vi "MainPanel_20170525.vi"() -> (0 "ErrorOut":errorcluster)   [LabVIEW 2018] (continued)
                n229 = call "LaunchSystemMessageDialogBox.vi"("ErrorToProcess"=w547, "SMS"=w542, "ErrorIn"=w549, "CorrAct"="Undocumented System Error, please record this information and contact the vendor.", "Timeout(ms)"=-1 ("Timeout (-1)")) -> ("ErrorOut"=w548:errorcluster)  [unwired: 6 in]
              }
              frame -8998 {
                # "-1 dictates that the message box does NOT time out"
                # "Default Error Case handles all error codes undefined by this structure."
                n230 = Bundle By Name(cluster=w553, "Stat.SysState"=SystemStateEnum."System Fault") -> (w552:T29)
                n231 = Unbundle By Name(w552) -> ("SMS"=w551:T33)
                n232 = call "LaunchSystemMessageDialogBox.vi"("ErrorToProcess"=w556, "SMS"=w551, "ErrorIn"=w558, "CorrAct"="The FPGAs are configured for an external 10 MHz reference clock. It doesn't look like that clock is working right.", "Timeout(ms)"=-1 ("Timeout (-1)")) -> ("ErrorOut"=w557:errorcluster)  [unwired: 6 in]
              }
              frame 5000 {
                # "Example User Defined Error Code.  Disable the Hardware and no Dialog Box"
                n233 = Bundle By Name(cluster=w560, "Stat.SysState"=SystemStateEnum."System Fault") -> (w561:T29)
              }
              frame 5998 {
                n234 = Unbundle By Name(w565) -> ("SMS"=w568:T33)
                n235 = call "LaunchSystemMessageDialogBox.vi"("ErrorToProcess"=w567, "SMS"=w568, "ErrorIn"=w564, "CorrAct"="Error Log Failure\n\n- There was an error writing to the Error Log File, please verify that the current user has read/write permissions to the <Users>\\My Documents & the <Users>\\Desktop folders" ("CorrAction"), "Timeout(ms)"=-1) -> ("ErrorOut"=w566:errorcluster)  [unwired: 6 in]
              }
              frame 5999 {
                n236 = Bundle By Name(cluster=w572, "Stat.SysState"=SystemStateEnum."System Error") -> (w573:T29)
              }
              frame 5100..5149 {
                # "Disable Hardware?"
                # "These error codes are reserved for Config File Reads"
                n237 = Bundle By Name(cluster=w582, "Stat.SysState"=SystemStateEnum."System Fault") -> (w576:T29)
                n238 = Unbundle By Name(w576) -> ("SMS"=w575:T33)
                n239 = call "LaunchSystemMessageDialogBox.vi"("ErrorToProcess"=w579, "SMS"=w575, "ErrorIn"=w578, "CorrAct"="Configuration File Read Error\n\n- One or more Configuration File Fields were not found or improperly loaded.\n- All System Hardware has been disabled\n- Launch the Configuration Panels and verify that all values have been correctly entered\n- Reinitialize the Hardware" ("CorrAction"), "Timeout(ms)"=-1 ("Timeout")) -> ("ErrorOut"=w577:errorcluster)  [unwired: 6 in]
              }
              frame 5150..5199 {
                # "No need to disable hardware here"
                # "These error codes are reserved for Config File Writes"
                n240 = Unbundle By Name(w584) -> ("SMS"=w585:T33)
                n241 = call "LaunchSystemMessageDialogBox.vi"("ErrorToProcess"=w588, "SMS"=w585, "ErrorIn"=w587, "CorrAct"="Configuration File Write Error\n\n- One or more Configuration File Fields were not found or specified incorrectly.\n- Launch the Configuration Panels and verify that all values have been correctly entered" ("CorrAction"), "Timeout(ms)"=-1 ("Timeout")) -> ("ErrorOut"=w586:errorcluster)  [unwired: 6 in]
              }
            }
          }
        }
      }
      frame "Spvsr_Config" {
        # "Opens the Configuration Panel"
        n242 = Current VI's Path() -> (path=w595:path)
        n243 = call "SetVIWindowTransparency.vi"("VIPath"=w595, "ErrorIn"=w596) -> ("ErrorOut"=w594:errorcluster)  [unwired: 9 in]
        n244 = call "ConfigPanel.vi"("ErrorIn"=w594, "ClusterIn"=w597) -> ("ErrorOut"=w590:errorcluster, "ClusterOut"=w591:T29)  [unwired: 8 out]
        n245 = Current VI's Path() -> (path=w592:path)
        n246 = call "RestoreVIWindowTransparency.vi"("VIPath"=w592, "ErrorIn"=w590) -> ("ErrorOut"=w593:errorcluster)  [unwired: 9 in]
      }
      frame "Spvsr_FPConfig" {
        w641 = ScaleMeasure."50" ("ScaleMeasure")
        w638 = ext 1.0 ("Scale_In_RT")
        w639 = fxp<+/-,30,30> 536870911.0 ("Scale_NoiseFloor")
        # "Don't start other loops if paths are bad."
        n247 = disable-structure shown="Enabled" {
          disable-tunnel: w603 -> [w661 _]
          disable-tunnel: [w660 T38 {"#NoiseSums"=1, "Max_df"=1, "AvgAvg"=FALSE, "#Avg"=1, "AutoCenter"=FALSE, "Inclin"={"Vmin"=0.0, "Vmax"=0.0, "Angle_min"=0.0, "Angle_max"=0.0, "Offset"=0.0, "Pos_Neg"=FALSE}, "1"={"Cal_"={"Fine"=0.000213623046875, "Coarse_"=4194303.0}, "Beac"={"Fine"=4194303.0, "Coarse_"=1.0}, "Scale"={"Step4"=10000.0, "Step5"=4194303.0, "Step6"=1.0, "Step7"=10000.0}, "Offset"=0.0, "Scale_Noise"=4194303.0, "Scale_Step1"=65535.0, "Scale_In_RT"=1.0, "ScaleMeas"=0.999969482421875, "FreqsToRemove"=[0, 1633], "Width"=[0, 1633], "ScaleMeasEnum"=enum."50", "FilterEnab"=enum."Step 1"}, "2"={"Cal_"={"Fine"=0.000213623046875, "Coarse_"=4194303.0}, "Beac"={"Fine"=0.000213623046875, "Coarse_"=4194303.0}, "Scale"={"Step4"=0.0, "Step5"=4194303.0, "Step6"=1.0, "Step7"=10000.0}, "Offset"=0.0, "Scale_Noise"=4194303.0, "Scale_Step1"=65535.0, "Scale_In_RT"=1.0, "ScaleMeas"=0.999969482421875, "FreqsToRemove"=[0, 1633], "Width"=[0, 1633], "ScaleMeasEnum"=enum."50", "FilterEnab"=enum."Step 1"}, "3"={"Cal_"={"Fine"=0.000213623046875, "Coarse_"=4194303.0}, "Beac"={"Fine"=0.000213623046875, "Coarse_"=4194303.0}, "Scale"={"Step4"=0.0, "Step5"=4194303.0, "Step6"=1.0, "Step7"=10000.0}, "Offset"=0.0, "Scale_Noise"=4194303.0, "Scale_Step1"=65535.0, "Scale_In_RT"=1.0, "ScaleMeas"=0.999969482421875, "FreqsToRemove"=[0, 1633], "Width"=[0, 1633], "ScaleMeasEnum"=enum."50", "FilterEnab"=enum."Step 1"}, "4"={"Cal_"={"Fine"=0.000213623046875, "Coarse_"=4194303.0}, "Beac"={"Fine"=0.000213623046875, "Coarse_"=4194303.0}, "Scale"={"Step4"=0.0, "Step5"=4194303.0, "Step6"=1.0, "Step7"=10000.0}, "Offset"=0.0, "Scale_Noise"=4194303.0, "Scale_Step1"=1.0, "Scale_In_RT"=10000.0, "ScaleMeas"=0.999969482421875, "FreqsToRemove"=[0, 1633], "Width"=[0, 1633], "ScaleMeasEnum"=enum."50", "FilterEnab"=enum."Step 1"}, "Target to Probe"=enum."4", "SNR_Thresh"=1.0, "Paths"={"CfgFile"=path "", "LogFolder"=path "", "LogFile"=path "", "NAS path"=path "", "ThreshFile"=path "", "RedunFolder"=path ""}, "Connex_Location"="", "SimulateFPGA"=FALSE, "Deadband"=0.0} ("FP_User")] -> w602
          frame Enabled {
            # "12/14/2020"
            n248 = Unbundle By Name(w661) -> ("Config.FP_User"=w660:T38)
          }
          frame Disabled {
          }
        }
        n249 = Unbundle By Name("Scale") -> ("Measure"=w625:fxp<+/-,16,1>, "Step1"=w626:fxp<+/-,17,17>, "Scale"=w627:T4)
        n250 = call "RootExists.vi"("path"="NAS path") -> ("file or folder exists?"=w605:bool)  [unwired: 10 in]
        n251 = Negate(x="Shift Cal") -> (-x=w620:T11)
        n252 = Negate(x="Shift Beac") -> (-x=w619:T11)
        n253 = Not(x=w605) -> (.not. x?=→"Logging to NAS":bool)
        n254 = Bundle By Name(cluster=w602, "1.ScaleMeas"=w625, "1.Scale_Step1"=w626, "1.Scale"=w627, "1.ScaleMeasEnum"=w641, "AvgAvg"="AvgAvg", "1.FreqsToRemove"="FreqsToRemove", "1.Width"="Width [bins]", "1.Cal_"=w620, "1.Beac"=w619, "1.FilterEnab"="FilterEnable", "1.Scale_Noise"=w639, "1.Scale_In_RT"=w638, "AutoCenter"="AutoCenter", "Target to Probe"="Target to Probe", "#Avg"=u16 150 ("#Avg in FPGA"), "SNR_Thresh"="SNR_Thresh", "Inclin"="Inclin", "Paths.RedunFolder"="base path", "Paths.LogFolder"="base path", "Paths.NAS path"="NAS path", "Paths.ThreshFile"="ThreshFile", "Connex_Location"="Location", "Max_df"="MaxTrackRate", "SimulateFPGA"="SimulateFPGA", "Deadband"="Deadband") -> (w650:T38)
        n255 = Build Array("base path", "ThreshFile") -> (w623:path[])
        n256 = Select(t=enum32{"Auto", "Manual"}."Auto" ("FreqShiftTab"), s="AutoCenter", f=enum32{"Auto", "Manual"}."Manual" ("FreqShiftTab")) -> (s? t:f=→"FreqShiftTab_72Co" →"FreqShiftTab_84Co":enum32{"Auto", "Manual"})
        n257 = for {
          tunnel: w623 -> [w672] mode=indexing
          tunnel: [w670] -> w622 mode=indexing
          n258 = call "RootDoesntExist.vi"("base path in"=w672) -> ("String"=w671:string)  [unwired: 10 in]
          n259 = call "RootExists.vi"("path"=w672) -> ("file or folder exists?"=w670:bool)  [unwired: 10 in]
          n260 = case shown="False" w670 {
            tunnel: w671 -> [w673 _]
            frame False {
              n261 = One Button Dialog(message=w673) -> ()  [unwired: 1 in, 1 out]
            }
            frame True {
            }
          }
        }
        n262 = Unbundle By Name(w650) -> ("2"=w649:T39)
        n263 = Bundle By Name(cluster=w649, "ScaleMeas"=w625, "Scale_Step1"=w626, "Scale"=w627, "ScaleMeasEnum"=w641, "FreqsToRemove"="FreqsToRemove", "Width"="Width [bins]", "FilterEnab"="FilterEnable", "Scale_Noise"=w639, "Scale_In_RT"=w638, "Cal_"=w620, "Beac"=w619) -> (w651:T39)
        n264 = Bundle By Name(cluster=w650, "2"=w651) -> (w644:T38)
        n265 = Negate(x="Shift Cal 3") -> (-x=w618:T11)
        n266 = Negate(x="Shift Beac 3") -> (-x=w617:T11)
        n267 = Unbundle By Name(w644) -> ("3"=w648:T39)
        n268 = Bundle By Name(cluster=w648, "ScaleMeas"=w625, "Scale_Step1"=w626, "Scale"=w627, "ScaleMeasEnum"=w641, "FreqsToRemove"="FreqsToRemove 2", "Width"="Width 2 [bins]", "FilterEnab"="FilterEnable", "Scale_Noise"=w639, "Scale_In_RT"=w638, "Cal_"=w618, "Beac"=w617) -> (w647:T39)
        n269 = And Array Elements(Boolean array=w622) -> (logical AND=w621:bool)
        n270 = Bundle By Name(cluster=w644, "3"=w647) -> (w643:T38)
        n271 = Unbundle By Name(w643) -> ("4"=w645:T39)
        n272 = Bundle By Name(cluster=w645, "ScaleMeas"=w625, "Scale_Step1"=w626, "Scale"=w627, "ScaleMeasEnum"=w641, "FreqsToRemove"="FreqsToRemove 2", "Width"="Width 2 [bins]", "FilterEnab"="FilterEnable", "Scale_Noise"=w639, "Scale_In_RT"=w638, "Cal_"=w618, "Beac"=w617) -> (w646:T39)
        n273 = Bundle By Name(cluster=w643, "4"=w646) -> (w642:T38)
        n274 = Bundle By Name(cluster=w603, "Config.FP_User"=w642) -> (w613:T29)
        n275 = Bundle By Name(cluster=w613, "Config.FP_User.Max_df"=u32 1) -> (w612:T29)
        n276 = case shown="True" w621 {
          tunnel: w659 -> [w663 w669]
          tunnel: w613 -> [_ w664]
          tunnel: w657 -> [_ w668]
          tunnel: [w663 w667] -> w653
          tunnel: w652 -> [_ w666]
          tunnel: w629 -> [_ w665]
          frame False {
          }
          frame True {
            n277 = call "Send_Front_Panel_Config_to_Loops.vi"("ClusterIn"=w664, "Log_Q"=w665, "error in (no error)"=w669, "Noise_Q"=w666, "Tones_Q"=w668) -> ("error out"=w667:errorcluster)  [unwired: 6 in]
          }
        }
        n278 = call "WriteConfigFile.vi"("ErrorIn"=w653, "ClusterIn"=w612) -> ("ErrorOut"=w658:errorcluster)  [unwired: 1 in, 8 out]
        "Auto Center" <- "AutoCenter"
      }
      frame "Spvsr_AlarmCfg" {
        # "We send alarm configurations to AI and TC. The voltage and\ntemp indicators are color-coded red & yellow if there are \nalarms or wanings. These are calculated in the AI loops."
        # "We need to send the alarm configuration to the log loop because that is\nwhere we will check the alarm statuses. It's the only place where we can find\nthe data from AI, TC, TE, ADAM, and spectra."
        n279 = Unbundle By Name(w686) -> ("Config.FP_User.Paths.ThreshFile"=w685:path)
        n280 = Bundle By Name(cluster=w686, "Alarm"="AlarmSettings") -> (w689:T29)
        n281 = Flatten To XML(anything="AlarmSettings") -> (xml string=w688:string)
        n282 = call-poly <vilib>:"Write to XML File.vi"("error in (no error)"=w687, "XML Input"=w688, "XML File Path"=w685) -> ("error out"=w684:errorcluster)  [unwired: 6 in, 2 out]
        n283 = To Variant(anything="AlarmSettings") -> (Variant=w675:variant)
        n284 = To Variant(anything="AlarmSettings") -> (Variant=w679:variant)
        n285 = Bundle By Name(cluster=cluster{"Enum":T17, "Data":variant} {"Enum"=enum."Log_CfgAlarm", "Data"=variant} ("element"), "Data"=w679) -> (w680:cluster{"Enum":T17, "Data":variant})
        n286 = Bundle By Name(cluster=cluster{"Enum":T49, "Var":variant} {"Enum"=enum."AI_Alarm", "Var"=variant}, "Var"=w675) -> (w676:cluster{"Enum":T49, "Var":variant})
        n287 = Enqueue Element(queue=w682, element=w680, error in (no error)=w684) -> (error out=w683:errorcluster)  [unwired: 1 in, 2 out]
        n288 = for {
          tunnel: string[] ["AI", "TC"] ("name (unnamed)") -> [w697] mode=indexing
          tunnel: w676 -> [w690]
          n289 = Obtain Queue(max queue size (-1, unlimited)=100, name (unnamed)=w697, element data type=w690) -> (queue out=w695:refnum<queue>, error out=w696:errorcluster)  [unwired: 2 in, 1 out]
          n290 = Enqueue Element(queue=w695, element=w690, error in (no error)=w696) -> (queue out=w693:refnum<queue>, error out=w694:errorcluster)  [unwired: 1 in, 1 out]
          n291 = Release Queue(queue=w693, error in (no error)=w694) -> (error out=w692:errorcluster)  [unwired: 1 in, 2 out]
          n292 = call "PushToErrorHandler.vi"("ErrorIn"=w692, "ErrorLocation"="SendAlarmToAI_orTC") -> ()  [unwired: 5 in, 1 out]
        }
      }
      frame "Spvsr_DigitzOffs" {
        w707 = fxp<+/-,16,16> 0.0 ("fixed-point type")
        n293 = local read "84 GHz"() -> (w715:T2)
        n294 = local read "72 GHz"() -> (w716:T2)
        n295 = Unbundle By Name(w716) -> ("MeasMean0"=w712:dbl, "MeasMean1"=w710:dbl)
        n296 = Unbundle By Name(w715) -> ("MeasMean0"=w709:dbl, "MeasMean1"=w708:dbl)
        n297 = Negate(x=w712) -> (-x=w702:dbl)
        n298 = Negate(x=w710) -> (-x=w701:dbl)
        n299 = Negate(x=w709) -> (-x=w700:dbl)
        n300 = Negate(x=w708) -> (-x=w699:dbl)
        n301 = To Fixed-Point(fixed-point type=w707, number=w702) -> (fixed-point=w711:fxp<+/-,16,16>)
        "Digitizer Offset 72 Co" <- w711
        n302 = To Fixed-Point(fixed-point type=w707, number=w701) -> (fixed-point=w705:fxp<+/-,16,16>)
        "Digitizer Offset 72 X" <- w705
        n303 = To Fixed-Point(fixed-point type=w707, number=w700) -> (fixed-point=w704:fxp<+/-,16,16>)
        "Digitizer Offset 84 Co" <- w704
        n304 = To Fixed-Point(fixed-point type=w707, number=w699) -> (fixed-point=w703:fxp<+/-,16,16>)
        "Digitizer Offset 84 x" <- w703
        n305 = Bundle By Name(cluster=w713, "Config.FP_User.1.Offset"=w711, "Config.FP_User.2.Offset"=w705, "Config.FP_User.3.Offset"=w704, "Config.FP_User.4.Offset"=w703) -> (w714:T29)
      }
      frame "FP_AO_ctrl" {
        w739 = 5.0
        w740 = 0.0
        w734 = cluster{"Enum":T51, "Data":variant} {"Enum"=enum."AO_Write", "Data"=variant}
        # "As defined in Wiring_Pinout Diagrams_DRAFT_20171207.xlsx\nfrom Nick Tarasenko.\nLuke 12-12-2017"
        # "Cal tones: 5 is on, 0 is off"
        # "Noise: 0 is on, 5 is off"
        n306 = Select(t=w740, s="noise_ctrl", f=w739) -> (s? t:f=w738:dbl)
        n307 = Select(t=w739, s="72GHz_ctrl", f=w740) -> (s? t:f=w737:dbl)
        n308 = Select(t=w739, s="84GHz_ctrl", f=w740) -> (s? t:f=w736:dbl)
        n309 = Obtain Queue(max queue size (-1, unlimited)=100, name (unnamed)="AO", element data type=w734, error in (no error)=w741) -> (queue out=w744:refnum<queue>, error out=w730:errorcluster)  [unwired: 1 in, 1 out]
        n310 = Build Array("noise_ctrl", "72GHz_ctrl", "84GHz_ctrl") -> (w719:bool[])
        n311 = Build Array(w738, w737, w736) -> (w735:dbl[])
        n312 = To Variant(anything=w735) -> (Variant=w723:variant)
        n313 = Bundle By Name(cluster=w734, "Data"=w723) -> (w733:cluster{"Enum":T51, "Data":variant})
        n314 = Enqueue Element(queue=w744, element=w733, error in (no error)=w730) -> (queue out=w729:refnum<queue>, error out=w731:errorcluster)  [unwired: 1 in, 1 out]
        n315 = To Variant(anything=w719) -> (Variant=w718:variant)
        n316 = Release Queue(queue=w729, error in (no error)=w731) -> (error out=w728:errorcluster)  [unwired: 1 in, 2 out]
        n317 = Bundle By Name(cluster=cluster{"Enum":T17, "Data":variant} {"Enum"=enum."Log_DO", "Data"=variant} ("element"), "Data"=w718) -> (w724:cluster{"Enum":T17, "Data":variant})
        n318 = Enqueue Element(queue=w726, element=w724, timeout in ms (-1)=10, error in (no error)=w728) -> (error out=w727:errorcluster)  [unwired: 2 out]
      }
      frame "Spvsr_ScaleGraphs" {
        w776 = 1000000.0 ("y")
        w773 = 10.0 ("y")
        n319 = local read "BeaconShift 3"() -> (w757:dbl)
        n320 = local read "BeaconShift 2"() -> (w789:dbl)
        n321 = local read "BeaconShift 4"() -> (w755:dbl)
        n322 = local read "BeaconShift"() -> (w785:dbl)
        n323 = local read "Peak Location Beacon"() -> (w771:dbl)
        n324 = local read "Peak Location Cal"() -> (w772:dbl)
        n325 = local read "Peak Location Beacon 2"() -> (w791:dbl)
        n326 = local read "Peak Location Cal 2"() -> (w792:dbl)
        n327 = local read "Peak Location Beacon 3"() -> (w753:dbl)
        n328 = local read "Peak Location Cal 3"() -> (w752:dbl)
        n329 = local read "Peak Location Beacon 4"() -> (w751:dbl)
        n330 = local read "Peak Location Cal 4"() -> (w750:dbl)
        n331 = local read "CalShift 3"() -> (w756:dbl)
        n332 = local read "CalShift 2"() -> (w790:dbl)
        n333 = local read "CalShift"() -> (w786:dbl)
        n334 = local read "CalShift 4"() -> (w754:dbl)
        n335 = control-ref of="NoiseFloor"() -> (w749:refnum<vi>)
        n336 = control-ref of="NoiseFloor 2"() -> (w747:refnum<vi>)
        n337 = control-ref of="NoiseFloor 3"() -> (w746:refnum<vi>)
        n338 = control-ref of="NoiseFloor 4"() -> (w745:refnum<vi>)
        n339 = local read "df (Hz)"() -> (w767:dbl)
        n340 = Build Array(w785, w786, w789, w790, w757, w756, w755, w754) -> (w780:dbl[])
        n341 = Build Array(w749, w747, w746, w745) -> (w748:refnum<vi>[])
        n342 = for {
          tunnel: [w820] -> w763
          tunnel: w780 -> [w822] mode=indexing
          tunnel: [w818] -> w762 mode=indexing
          n343 = local read "df (Hz)"() -> (w823:dbl)
          n344 = Divide(x=w823, y=1000000.0) -> (x/y=w820:dbl)
          n345 = Divide(x=w822, y=1000000.0) -> (x/y=w818:dbl)
        }
        n346 = Build Array(w771, w772, w791, w792, w753, w752, w751, w750) -> (w781:dbl[])
        n347 = for {
          tunnel: w767 -> [w795]
          tunnel: u8 0 ("Noise Floor") -> [w794]
          tunnel: w748 -> [w793] mode=indexing
          n348 = property class="WFGraph (strict)"(reference=w793, "YScale.Mapping Mode"=w794, "XScale.Multiplier"=w795) -> ()  [unwired: 1 in, 2 out]
        }
        n349 = case shown="True" "AutoScale Y Noise" {
          tunnel: w748 -> [_ w796]
          frame False {
          }
          frame True {
            n350 = for {
              tunnel: w796 -> [w798] mode=indexing
              n351 = property class="WFGraph (strict)"(reference=w798, "YScale.ScaleFit"=u8 1 ("Y Scale.Scale Fit")) -> ()  [unwired: 1 in, 2 out]
            }
          }
        }
        n352 = Add(x=w781, y=w773) -> (x+y=w774:dbl[])
        n353 = Subtract(x=w781, y=w773) -> (x-y=w775:dbl[])
        n354 = Divide(x=w774, y=w776) -> (x/y=w778:dbl[])
        n355 = Divide(x=w775, y=w776) -> (x/y=w779:dbl[])
        n356 = control-ref of="Beacon 2"() -> (w787:refnum<vi>)
        n357 = control-ref of="Cal 2"() -> (w788:refnum<vi>)
        n358 = control-ref of="Beacon 3"() -> (w761:refnum<vi>)
        n359 = control-ref of="Beacon"() -> (w770:refnum<vi>)
        n360 = control-ref of="Cal"() -> (w768:refnum<vi>)
        n361 = control-ref of="Cal 3"() -> (w760:refnum<vi>)
        n362 = control-ref of="Cal 4"() -> (w758:refnum<vi>)
        n363 = control-ref of="Beacon 4"() -> (w759:refnum<vi>)
        n364 = Build Array(w770, w768, w787, w788, w761, w760, w759, w758) -> (w782:refnum<vi>[])
        n365 = for {
          tunnel: w782 -> [w827] mode=indexing
          tunnel: u8 0 ("Tones") -> [w826]
          tunnel: w763 -> [w825]
          tunnel: w762 -> [w824] mode=indexing
          n366 = property class="WFGraph"(reference=w827, "YScale.Mapping Mode"=w826, "XScale.Multiplier"=w825, "XScale.Offset"=w824) -> ()  [unwired: 1 in, 2 out]
        }
        n367 = for {
          tunnel: w782 -> [w806] mode=indexing
          tunnel: "Zoom On Peak" -> [w805]
          tunnel: w778 -> [w804] mode=indexing
          tunnel: w779 -> [w803] mode=indexing
          tunnel: [w802] -> _
          n368 = case shown="True" w805 {
            tunnel: w806 -> [w811 w813]
            tunnel: w804 -> [w809 _]
            tunnel: w803 -> [w808 _]
            tunnel: [w807 w812] -> w802
            frame True {
              n369 = property class="WFGraph"(reference=w811, "XScale.ScaleFit"=u8 0 ("X Scale.Scale Fit"), "XScale.Maximum"=w809, "XScale.Minimum"=w808) -> (error out=w807:errorcluster)  [unwired: 1 in, 1 out]
            }
            frame False {
              n370 = disable-structure shown="Disabled" {
                disable-tunnel: w813 -> [w816 _]
                disable-tunnel: [w814 errorcluster {"status"=FALSE, "code"=0, "source"=""} ("error out")] -> w812
                frame Enabled {
                  n371 = property class="WFGraph"(reference=w816, "XScale.ScaleFit"=u8 2 ("X Scale.Scale Fit")) -> (error out=w814:errorcluster)  [unwired: 1 in, 1 out]
                }
                frame Disabled {
                }
              }
            }
          }
        }
        n372 = case shown="True" "AutoScale Y Tones" {
          tunnel: w782 -> [_ w799]
          frame False {
          }
          frame True {
            n373 = for {
              tunnel: w799 -> [w800] mode=indexing
              n374 = property class="WFGraph"(reference=w800, "YScale.ScaleFit"=u8 1 ("Y Scale.Scale Fit")) -> ()  [unwired: 1 in, 2 out]
            }
          }
        }
      }
      frame "Spvsr_TrackRate" {
        n375 = Bundle By Name(cluster=w829, "Stat.TrackRate"=FALSE) -> (w830:T29)
      }
      frame "Spvsr_AutoCenter" {
        w832 = FALSE  # Stat.AutoCentr
        n376 = Bundle By Name(cluster=w833, "Stat.AutoCentr"=w832) -> (w834:T29)
      }
      frame "Spvsr_RestartWarn" {
        n377 = One Button Dialog(message="When changing file paths, the change will not be implemented until the program is restarted.\n\nWhen changing the \"Connex Location\", the change will not be written to the data log header until a new file is made (either at midnight, or upon restarting.)") -> ()  [unwired: 1 in, 1 out]
      }
      frame "Spvsr_ChkTime" {
        # "Reset peak tracker to default 10 minutes after user changes it."
        # "Variable is updated in Log_TCP"
        n378 = Unbundle By Name(w854) -> ("Stat.AutoCentr"=w846:bool, "Stat.TrackRate"=w856:bool)
        n379 = call "Elapsed Time4"("Time Target (s)"=600.0, "Reset"=w856, "error in (no error)"=w857) -> ("Elapsed Time (s)"=w852:dbl, "Time has Elapsed"=w855:bool, "error out"=w853:errorcluster)  [unwired: 9 in, 5 out]
        n380 = case shown="True" w855 {
          tunnel: w854 -> [w875 w883]
          tunnel: [w875 w882] -> w843
          tunnel: w853 -> [w876 w880]
          tunnel: [w876 w877] -> w845
          tunnel: w852 -> [_ _]
          frame False {
          }
          frame True {
            n381 = control-ref of="MaxTrackRate"() -> (w879:refnum<vi>)
            n382 = property class="DigNum (strict)"(reference=w879, error in=w880, "Val(Sgnl)"=u32 1 ("Value (Signaling)")) -> (error out=w877:errorcluster)  [unwired: 1 out]
            n383 = Bundle By Name(cluster=w883, "Stat.TrackRate"=TRUE) -> (w882:T29)
          }
        }
        n384 = call "Elapsed Time5"("Time Target (s)"=600.0, "Reset"=w846, "error in (no error)"=w845) -> ("Elapsed Time (s)"=w849:dbl, "Time has Elapsed"=w847:bool, "error out"=w848:errorcluster)  [unwired: 9 in, 5 out]
        n385 = case shown="True" w847 {
          tunnel: w843 -> [w866 w874]
          tunnel: [w866 w873] -> w842
          tunnel: w848 -> [w867 w871]
          tunnel: [w867 w869] -> w844
          tunnel: w849 -> [_ _]
          frame False {
          }
          frame True {
            n386 = control-ref of="AutoCenter"() -> (w870:refnum<vi>)
            n387 = property class="Bool (strict)"(reference=w870, error in=w871, "Val(Sgnl)"=TRUE ("Value (Signaling)")) -> (error out=w869:errorcluster)  [unwired: 1 out]
            n388 = Bundle By Name(cluster=w874, "Stat.AutoCentr"=TRUE ("Stat.TrackRate")) -> (w873:T29)
          }
        }
        n389 = shared-variable ".\\Connex_Variables.lvlib\\TCP_Status"() -> (→"TCP Connection":bool)  [unwired: 1 in, 1 out]
        n390 = call "Elapsed Time3"("Time Target (s)"=2.0, "error in (no error)"=w844) -> ("Time has Elapsed"=w863:bool, "error out"=w840:errorcluster)  [unwired: 10 in, 6 out]
        n391 = Select(t=cluster{"QElmnt":T44, "Data":variant}[] [{"QElmnt"=enum."Spvsr_ScaleGraphs", "Data"=variant}, {"QElmnt"=enum."Spvsr_ChkTime", "Data"=variant}], s=w863, f=cluster{"QElmnt":T44, "Data":variant}[] [{"QElmnt"=enum."Spvsr_ChkTime", "Data"=variant}]) -> (s? t:f=w865:cluster{"QElmnt":T44, "Data":variant}[])
        n392 = for {
          tunnel: w865 -> [w886] mode=indexing
          tunnel: w864 -> [w885]
          shift-right: [w884] -> w860
          shift-left: _ -> [_]
          n393 = Enqueue Element(queue=w885, element=w886) -> (error out=w884:errorcluster)  [unwired: 2 in, 2 out]
        }
        n394 = Wait Until Next ms Multiple(millisecond multiple=u32 100 ("milliseconds to wait")) -> ()  [unwired: 1 out]
        n395 = Merge Errors(w860, w840) -> (w841:errorcluster)
      }
      frame "Spvsr_About" {
        # "Pops up the About dialog box where you can enter version, customer, contact and any other information regarding the application."
        n396 = call "About.vi"("error in"=w890, "Timeout (ms)"=5000) -> ("error out"=w889:errorcluster)  [unwired: 9 out]
      }
      frame "Spvsr_Exit" {
        # "With the Exit Button, we exit this loop and push the HW Loops to close."
        n397 = call "Exit_All_Loops.vi"("error in (no error)"=w892, "10Hz_Q"=w891, "Noise_Q"=w894, "Tones_Q"=w895) -> ("error out"=w893:errorcluster)  [unwired: 7 in]
      }
    }
    "SPVSR_Count" <- w285
  }
  n398 = call "PXI_Health_Loop.vi"("error in (no error)"=w1) -> ("error out"=w117:errorcluster)  [unwired: 10 in]
  n399 = while {
    tunnel: w77 -> [w899]
    tunnel: w100 -> [w909]
    tunnel: [w903] -> w137
    shift-right: [w902] -> _
    shift-left: T20 {"Alarms"={"Green"=FALSE, "Rx_Yell"=FALSE, "Cx_Yell"=FALSE, "Red"=FALSE, "Source"=""}, "Spectrum 1"=[], "Spectrum 2"=[], "Spectrum 3"=[], "Spectrum 4"=[], "HistoryWeighting"=0.0, "NoiseFloorSums"={"1"=0.0, "2"=0.0, "3"=0.0, "4"=0.0}, "PwrHist"={"72Co"={"Cal"=0.0, "Cal Smooth"=0.0, "Beac"=0.0, "Beac Smooth"=0.0, "NoiseFloorSum"=0.0, "NoiseFloorSum Smooth"=0.0}, "72X"={"Cal"=0.0, "Cal Smooth"=0.0, "Beac"=0.0, "Beac Smooth"=0.0, "NoiseFloorSum"=0.0, "NoiseFloorSum Smooth"=0.0}, "84Co"={"Cal"=0.0, "Cal Smooth"=0.0, "Beac"=0.0, "Beac Smooth"=0.0, "NoiseFloorSum"=0.0, "NoiseFloorSum Smooth"=0.0}, "84X"={"Cal"=0.0, "Cal Smooth"=0.0, "Beac"=0.0, "Beac Smooth"=0.0, "NoiseFloorSum"=0.0, "NoiseFloorSum Smooth"=0.0}}} -> [w901]
    i -> [w900]
    stop <- w904 stop-if-true
    # "Front panel updates"
    n400 = call "PushToErrorHandler.vi"("ErrorIn"=w909, "ErrorLocation"="FP") -> ("ErrorOut"=w911:errorcluster)  [unwired: 5 in]
    n401 = Get Queue Status(queue=w899) -> (# elements in queue=→"# in FP queue":i32)  [unwired: 2 in, 7 out]
    n402 = Dequeue Element(queue=w899, error in (no error)=w911) -> (queue out=w905:refnum<queue>, element=w910:cluster{"Enum":T26, "Data":variant}, error out=w906:errorcluster)  [unwired: 1 in, 1 out]
    n403 = Unbundle(w910) -> ("Enum"=w908:T26, "Data"=w907:variant)
    n404 = case shown="\"FP_Tone\"" w908 {
      tunnel: w907 -> [_ _ w930 w1074 w1123 w1133 w1153 w1164 _ w1251 _]
      tunnel: w906 -> [w916 w918 w923 w1075 w1125 w1135 w1155 w1165 w1180 w1252 w1264]
      tunnel: w905 -> [_ _ w921 _ _ _ _ _ _ _ w1265]
      tunnel: [_ _ _ _ _ _ _ _ _ _ TRUE] -> w904
      tunnel: [w916 w918 w923 w1075 w1126 w1134 w1154 w1159 w1180 w1240 w1263] -> w903
      tunnel: [w917 w919 w924 w1068 w1112 w1127 w1146 w1160 w1179 w1181 w1262] -> w902
      tunnel: w901 -> [w917 w919 w925 w1069 w1112 w1127 w1146 w1160 w1179 w1181 w1262]
      frame "FP_Init", Default {
        w915 = cluster{dbl, dbl, dbl}[] [] ("History Data")
        n405 = control-ref of="Freq History 84 Co"() -> (w913:refnum<vi>)
        n406 = control-ref of="Freq History 72 Co"() -> (w914:refnum<vi>)
        n407 = property class="WFChart (strict)"(reference=w914, "History Data"=w915) -> ()  [unwired: 1 in, 2 out]
        n408 = property class="WFChart (strict)"(reference=w913, "History Data"=w915) -> ()  [unwired: 1 in, 2 out]
      }
      frame "FP_Scale" {
      }
      frame "FP_Tone" {
        # "From Data_Send"
        n409 = local read "SNR_Thresh"() -> (w920:dbl)
        n410 = local read "AutoCenter"() -> (w922:bool)
        n411 = Variant To Data(error in=w923, type=cluster{"Target":T16, "1":T52} {"Target"=enum."1", "1"={"Cal"={"Shift_"=0.0, "Peak_ToFPGA"=-24999462.633451957, "MaxValue"=0.0, "MaxIndex"=0, "Tone"={"PkLocTrak"=0.0, "PkLocDisp"=0.0, "df_"=0.0, "ZoomPwr"=[], "Phase"=0.0, "PhaseOld"=0.0, "AboveThresh?"=FALSE, "MaxI"=0.0, "MaxQ"=0.0, "median"=0.0, "ISpect"=[], "QSpect"=[], "DeltaPhase"=0.0}, "TimeDomainI"=[], "TimeDomainQ"=array[12500 elements], "PwrSpectrum"=[], "RunningAvgFreq"=0.0, "ISpectPos"=[], "ISpectNeg"=[], "QSpectPos"=[], "QSpectNeg"=[], "10Hz_PwrSpectr"=[], "SNR"=0.0, "AliasWarn"=FALSE, "10Hz_Peak"=[], "ISpect+-"=[], "QSpect+-"=[], "TimeStamp"=timestamp(0 s since 1904-01-01), "I_Index"=array[12500 elements], "Q_Index"=array[12500 elements], "10MHz"=FALSE}, "Beac"={"Shift_"=0.0, "Peak_ToFPGA"=-24999462.633451957, "MaxValue"=0.0, "MaxIndex"=0, "Tone"={"PkLocTrak"=0.0, "PkLocDisp"=0.0, "df_"=0.0, "ZoomPwr"=[], "Phase"=0.0, "PhaseOld"=0.0, "AboveThresh?"=FALSE, "MaxI"=0.0, "MaxQ"=0.0, "median"=0.0, "ISpect"=[], "QSpect"=[], "DeltaPhase"=0.0}, "TimeDomainI"=[], "TimeDomainQ"=array[12500 elements], "PwrSpectrum"=[], "RunningAvgFreq"=0.0, "ISpectPos"=[], "ISpectNeg"=[], "QSpectPos"=[], "QSpectNeg"=[], "10Hz_PwrSpectr"=[], "SNR"=0.0, "AliasWarn"=FALSE, "10Hz_Peak"=[], "ISpect+-"=[], "QSpect+-"=[], "TimeStamp"=timestamp(0 s since 1904-01-01), "I_Index"=array[12500 elements], "Q_Index"=array[12500 elements], "10MHz"=FALSE}, "Time"=[], "Saturat"={"MeasMean0"=0.0, "MeasMean1"=0.0, "MeasMax"=0.0, "1_Max"=0.0, "4_Max"=0.0, "5_Max"=0.0, "6_Max"=0.0, "7_Max"=0.0}}} ("cluster"), Variant=w930) -> (data=w928:cluster{"Target":T16, "1":T52})  [unwired: 1 out]
        n412 = Unbundle(w928) -> ("Target"=w927:T16, "1"=w926:T52)
        n413 = case shown="\"2\", Default" w927 {
          tunnel: w926 -> [w970 w997 w1035 w1064]
          tunnel: w925 -> [w960 w985 w1021 w1051]
          tunnel: [w961 w989 w1028 w1057] -> w924
          tunnel: w922 -> [w956 _ w1024 _]
          tunnel: w921 -> [_ _ _ w1038]
          tunnel: w920 -> [w946 _ w1017 _]
          frame "1" {
            # "Reset\nWatchdog"
            # "Update all history charts"
            # "All freq locations displayed as positive."
            # "df is the same for cal & beac"
            n414 = Unbundle By Name(w970) -> ("Cal"=w969:T53, "Saturat"=→"72 GHz":T2, "Beac"=w967:T53)
            n415 = Unbundle By Name(w967) -> ("Shift_"=w966:dbl, "MaxValue"=w954:dbl, "Tone"=w945:T54, "TimeDomainI"=→"TimeDomainBeac 72Co":ext[], "PwrSpectrum"=w948:dbl[], "SNR"=→"SNR":dbl)
            "Channel Power Beac" <- w954
            n416 = Unbundle By Name(w969) -> ("Shift_"=w968:dbl, "MaxValue"=w941:dbl, "Tone"=w952:T54, "TimeDomainI"=→"TimeDomainCal 72Co":ext[], "PwrSpectrum"=→"Cal":dbl[])
            "Channel Power Cal" <- w941
            "MaxValue_Cal_72Co" <- w941
            n417 = Unbundle By Name(w945) -> ("PkLocDisp"=w964:dbl)
            n418 = Negate(x=w968) -> (-x=w942:dbl)
            "CalShift" <- w942
            n419 = Negate(x=w966) -> (-x=w944:dbl)
            "BeaconShift" <- w944
            n420 = Unbundle By Name(w952) -> ("PkLocTrak"=w965:dbl, "df_"=→"df (Hz)":dbl)
            n421 = Negate(x=w964) -> (-x=w943:dbl)
            "Peak Location Beacon" <- w943
            n422 = Unbundle By Name(w945) -> ("median"=w949:dbl, "Phase"=→"72 Co Beac":dbl)
            n423 = Negate(x=w965) -> (-x=w934:dbl)
            "Peak Location Cal" <- w934
            n424 = call "CombineSpectrumAndMedian.vi"("SNR_Thresh"=w946, "median"=w949, "PwrSpectrum"=w948) -> ("Array"=→"Beacon":dbl[][])  [unwired: 8 in]
            n425 = Bundle(w934, w943, w944) -> (→"Freq History 72 Co":cluster{dbl, dbl, dbl})  [unwired: 1 in]
            n426 = local read "NoiseFloorSum"() -> (w959:dbl)
            n427 = Divide(x=w934, y=1000000.0 ("x")) -> (x/y=→"72CoCalFrq":dbl)
            n428 = Divide(x=w943, y=1000000.0 ("x")) -> (x/y=→"72CoBeacFrq":dbl)
            n429 = call "BuildHistoryCluster.vi"("NewValueWeighting"="NewValueWeighting", "NoiseFloorSum"=w959, "Channel Power Beac"=w954, "Channel Power Cal"=w941) -> ("output cluster"=w933:T68)  [unwired: 7 in]
            n430 = control-ref of="Shift Beac"() -> (w957:refnum<vi>)
            n431 = control-ref of="Shift Cal"() -> (w958:refnum<vi>)
            n432 = Bundle By Name(cluster=w960, "Spectrum 1"=w948, "HistoryWeighting"="NewValueWeighting", "PwrHist.72Co"=w933) -> (w961:T20)
            n433 = call "OverWriteManualShiftValues.vi"("AutoCenter"=w956, "Shift Beac Val"=w944, "Shift Beac Ref"=w957, "Shift Cal Val"=w942, "Shift Cal Ref"=w958) -> ()  [unwired: 7 in]
            n434 = call "Watchdog_Functional_Global.vi"("Watchdog"=WatchdogTimer_Enum."FP") -> ()  [unwired: 8 in, 3 out]
          }
          frame "2", Default {
            n435 = Unbundle By Name(w997) -> ("Cal"=w996:T53, "Beac"=w995:T53)
            n436 = Unbundle By Name(w995) -> ("Shift_"=w994:dbl, "MaxValue"=w987:dbl, "Tone"=w982:T54, "TimeDomainI"=→"TimeDomainBeacon 72 X":ext[], "PwrSpectrum"=w988:dbl[], "SNR"=→"SNR 2":dbl, "Tone.DeltaPhase"=→"Delta Phase 72 GHz":dbl)
            "Beacon 2" <- w988
            "Channel Power Beac 2" <- w987
            n437 = Unbundle By Name(w996) -> ("Shift_"=w993:dbl, "MaxValue"=w974:dbl, "Tone"=w983:T54, "TimeDomainI"=→"TimeDomainCal 72 X":ext[], "PwrSpectrum"=→"Cal 2":dbl[])
            "Channel Power Cal 2" <- w974
            "MaxValue_Cal_72X" <- w974
            n438 = Unbundle By Name(w983) -> ("PkLocTrak"=w991:dbl)  [unwired: 1 out]
            n439 = Negate(x=w993) -> (-x=→"CalShift 2":dbl)
            n440 = Unbundle By Name(w982) -> ("PkLocDisp"=w992:dbl)
            n441 = Negate(x=w994) -> (-x=→"BeaconShift 2":dbl)
            n442 = Unbundle By Name(w982) -> ("Phase"=→"72 X Beac":dbl)
            n443 = Negate(x=w991) -> (-x=→"Peak Location Cal 2":dbl)
            n444 = Negate(x=w992) -> (-x=→"Peak Location Beacon 2":dbl)
            n445 = Unbundle By Name(w985) -> ("HistoryWeighting"=w984:dbl)
            n446 = local read "NoiseFloorSum 2"() -> (w986:dbl)
            n447 = call "BuildHistoryCluster.vi"("NewValueWeighting"=w984, "NoiseFloorSum"=w986, "Channel Power Beac"=w987, "Channel Power Cal"=w974) -> ("output cluster"=w971:T68)  [unwired: 7 in]
            n448 = Bundle By Name(cluster=w985, "Spectrum 2"=w988, "PwrHist.72X"=w971) -> (w989:T20)
          }
          frame "3" {
            # "Disdrometer device resets every 90 days UNLESS signal is too low. Using a variable\nbecause there is no other mechanism for sending data to Disdrometer"
            n449 = Unbundle By Name(w1035) -> ("Cal"=w1034:T53, "Saturat"=→"84 GHz":T2, "Beac"=w1010:T53)
            n450 = Unbundle By Name(w1010) -> ("Shift_"=w1033:dbl, "MaxValue"=w1023:dbl, "Tone"=w1014:T54, "TimeDomainI"=→"TimeDomain Beac 84 Co":ext[], "PwrSpectrum"=w1018:dbl[], "SNR"=w1012:dbl)
            "Channel Power Beac 3" <- w1023
            "SNR 3" <- w1012
            n451 = Unbundle By Name(w1034) -> ("Shift_"=w1032:dbl, "MaxValue"=w1011:dbl, "Tone"=w1019:T54, "TimeDomainI"=→"TimeDomainCal 84 Co":ext[], "PwrSpectrum"=→"Cal 3":dbl[])  [unwired: 1 out]
            "Channel Power Cal 3" <- w1011
            "MaxValue_Cal_84Co" <- w1011
            n452 = Unbundle By Name(w1014) -> ("PkLocDisp"=w1031:dbl)
            n453 = Unbundle By Name(w1014) -> ("Phase"=→"84 Co Beac":dbl, "median"=w1016:dbl)
            n454 = Unbundle By Name(w1019) -> ("PkLocTrak"=w1030:dbl)  [unwired: 1 out]
            n455 = Negate(x=w1033) -> (-x=w1013:dbl)
            "BeaconShift 3" <- w1013
            n456 = Negate(x=w1032) -> (-x=w1027:dbl)
            "CalShift 3" <- w1027
            n457 = Negate(x=w1031) -> (-x=w1004:dbl)
            "Peak Location Beacon 3" <- w1004
            n458 = Negate(x=w1030) -> (-x=w1002:dbl)
            "Peak Location Cal 3" <- w1002
            n459 = shared-variable ".\\Disdrometer_Vars.lvlib\\Disdrom_SNR"(w1012) -> ()  [unwired: 1 in, 1 out]
            n460 = Divide(x=w1002, y=1000000.0 ("x")) -> (x/y=→"84CoCalFrq":dbl)
            n461 = call "CombineSpectrumAndMedian.vi"("SNR_Thresh"=w1017, "median"=w1016, "PwrSpectrum"=w1018) -> ("Array"=→"Beacon 3":dbl[][])  [unwired: 8 in]
            n462 = Divide(x=w1004, y=1000000.0 ("x")) -> (x/y=→"84CoBeacFrq":dbl)
            n463 = Bundle(w1002, w1004, w1013) -> (→"Freq History 84 Co":cluster{dbl, dbl, dbl})  [unwired: 1 in]
            n464 = local read "NoiseFloorSum 2"() -> (w1022:dbl)
            n465 = Unbundle By Name(w1021) -> ("HistoryWeighting"=w1020:dbl)
            n466 = call "BuildHistoryCluster.vi"("NewValueWeighting"=w1020, "NoiseFloorSum"=w1022, "Channel Power Beac"=w1023, "Channel Power Cal"=w1011) -> ("output cluster"=w999:T68)  [unwired: 7 in]
            n467 = control-ref of="Shift Cal 3"() -> (w1026:refnum<vi>)
            n468 = control-ref of="Shift Beac 3"() -> (w1025:refnum<vi>)
            n469 = Bundle By Name(cluster=w1021, "Spectrum 3"=w1018, "PwrHist.84Co"=w999) -> (w1028:T20)
            n470 = call "OverWriteManualShiftValues.vi"("AutoCenter"=w1024, "Shift Beac Val"=w1013, "Shift Beac Ref"=w1025, "Shift Cal Val"=w1027, "Shift Cal Ref"=w1026) -> ()  [unwired: 7 in]
          }
          frame "4" {
            n471 = Unbundle By Name(w1064) -> ("Cal"=w1063:T53, "Beac"=w1062:T53)
            n472 = Unbundle By Name(w1062) -> ("Shift_"=w1061:dbl, "MaxValue"=w1053:dbl, "Tone"=w1048:T54, "TimeDomainI"=→"TimeDomainBeacon 84 X":ext[], "PwrSpectrum"=w1055:dbl[], "SNR"=→"SNR 4":dbl, "Tone.DeltaPhase"=→"Delta Phase 84 GHz":dbl)
            "Beacon 4" <- w1055
            "Channel Power Beac 4" <- w1053
            n473 = Unbundle By Name(w1063) -> ("Shift_"=w1060:dbl, "MaxValue"=w1041:dbl, "Tone"=w1049:T54, "TimeDomainI"=→"TimeDomainCal 84 X":ext[], "PwrSpectrum"=→"Cal 4":dbl[])
            "Channel Power Cal 4" <- w1041
            "MaxValue_Cal_84X" <- w1041
            n474 = Unbundle By Name(w1048) -> ("Phase"=→"84 X Beac":dbl)
            n475 = Negate(x=w1061) -> (-x=→"BeaconShift 4":dbl)
            n476 = Unbundle By Name(w1048) -> ("PkLocDisp"=w1059:dbl)
            n477 = Unbundle By Name(w1049) -> ("PkLocTrak"=w1058:dbl)
            n478 = Negate(x=w1060) -> (-x=→"CalShift 4":dbl)
            n479 = Negate(x=w1059) -> (-x=→"Peak Location Beacon 4":dbl)
            n480 = Negate(x=w1058) -> (-x=→"Peak Location Cal 4":dbl)
            n481 = Unbundle By Name(w1051) -> ("HistoryWeighting"=w1050:dbl)
            n482 = local read "NoiseFloorSum 2"() -> (w1052:dbl)
            n483 = call "BuildHistoryCluster.vi"("NewValueWeighting"=w1050, "NoiseFloorSum"=w1052, "Channel Power Beac"=w1053, "Channel Power Cal"=w1041) -> ("output cluster"=w1037:T68)  [unwired: 7 in]
            n484 = Bundle By Name(cluster=w1051, "Spectrum 4"=w1055, "PwrHist.84X"=w1037) -> (w1057:T20)
            n485 = for {
              tunnel: w1038 -> [w1067]
              tunnel: cluster{"Enum":T26, "Data":variant}[] [{"Enum"=enum."FP_Scale", "Data"=variant}, {"Enum"=enum."FP_PWR_Hist", "Data"=variant}] ("element") -> [w1066] mode=indexing
              n486 = Enqueue Element(queue=w1067, element=w1066, timeout in ms (-1)=10) -> ()  [unwired: 1 in, 3 out]
            }
          }
        }
      }
      frame "FP_Noise" {
        # "From Noise_Send"
        n487 = Variant To Data(error in=w1075, type=cluster{"Target":T16, "1":T55} {"Target"=enum."1", "1"={"df"=0.0, "AvgAvgSpectrum"=[], "FFT_Index"=[], "Avg'd"=[], "Sum"=0.0, "SumdSpectrum"=[], "SumCount"=0, "DayOfYear"=0}} ("cluster"), Variant=w1074) -> (data=w1073:cluster{"Target":T16, "1":T55})  [unwired: 1 out]
        n488 = Unbundle(w1073) -> ("Target"=w1072:T16, "1"=w1071:T55)
        n489 = case shown="\"4\"" w1072 {
          tunnel: w1071 -> [w1082 w1087 w1092 w1097]
          tunnel: w1069 -> [w1079 w1085 w1090 w1095]
          tunnel: [w1077 w1084 w1089 w1094] -> w1068
          frame "1", Default {
            n490 = Unbundle By Name(w1082) -> ("df"=→"df (Hz)":dbl, "AvgAvgSpectrum"=→"NoiseFloor":dbl[], "Sum"=w1078:dbl)  [unwired: 2 out]
            "NoiseFloorSum" <- w1078
            n491 = Bundle By Name(cluster=w1079, "NoiseFloorSums.1"=w1078) -> (w1077:T20)
            n492 = Unbundle By Name(w1077) -> ("NoiseFloorSums"=→"Noise Floor Sum Histories":T22)
          }
          frame "2" {
            n493 = Unbundle By Name(w1087) -> ("AvgAvgSpectrum"=→"NoiseFloor 2":dbl[], "Sum"=w1083:dbl)  [unwired: 3 out]
            "NoiseFloorSum 2" <- w1083
            n494 = Bundle By Name(cluster=w1085, "NoiseFloorSums.2"=w1083) -> (w1084:T20)
          }
          frame "3" {
            n495 = Unbundle By Name(w1092) -> ("AvgAvgSpectrum"=→"NoiseFloor 3":dbl[], "Sum"=w1088:dbl)  [unwired: 3 out]
            "NoiseFloorSum 3" <- w1088
            n496 = Bundle By Name(cluster=w1090, "NoiseFloorSums.3"=w1088) -> (w1089:T20)
          }
          frame "4" {
            n497 = Unbundle By Name(w1097) -> ("AvgAvgSpectrum"=→"NoiseFloor 4":dbl[], "Sum"=w1093:dbl)  [unwired: 3 out]
            "NoiseFloorSum 4" <- w1093
            n498 = Bundle By Name(cluster=w1095, "NoiseFloorSums.4"=w1093) -> (w1094:T20)
          }
        }
      }
      frame "FP_Probes" {
        n499 = Variant To Data(error in=w1125, type=T56 {"Probe 1"=0, "Probe 2"=0.0, "Probe 3"=0.0, "Probe 4"=0.0, "Probe 5"=0.0, "Probe 6"=0.0, "Probe 7"=0.0, "Probe 7_1"=0.0, "IProbe"={"Probe 8"=0.0, "Probe 9"=0.0, "Probe 10"=0.0, "Probe 11"=0.0, "Probe 12"=0.0, "Probe 13"=0.0, "Probe 14"=0.0, "Probe 15"=0.0, "Probe 16"=0.0, "Probe 17"=0.0, "Probe 18"=0.0, "Probe 19"=0.0, "Probe20"=0.0}, "Probe 21"=0.0, "Probe 22"=0.0, "Probe 23"=0.0, "Probe 24"=0.0, "Probe Offsetd"=0.0, "CalShiftProbe"=0.0, "QProbe"={"Probe 8"=0.0, "Probe 9"=0.0, "Probe 10"=0.0, "Probe 11"=0.0, "Probe 12"=0.0, "Probe 13"=0.0, "Probe 14"=0.0, "Probe 15"=0.0, "Probe 16"=0.0, "Probe 17"=0.0, "Probe 18"=0.0, "Probe 19"=0.0, "Probe20"=0.0}, "AI_Over"=FALSE, "10MHzLocked"=FALSE} ("FPGA_Probes"), Variant=w1123) -> (data=w1122:T56, error out=w1126:errorcluster)
        n500 = shared-variable ".\\Connex_Variables.lvlib\\FAM Init 1"() -> (→"Digitizer 1 Init Attempts":i32)  [unwired: 1 in, 1 out]
        n501 = shared-variable ".\\Connex_Variables.lvlib\\FAM Init 2"() -> (→"Digitizer 2 Init Attempts":i32)  [unwired: 1 in, 1 out]
        n502 = Unbundle By Name(w1122) -> ("Probe 1"=→"Probe 1":i16, "Probe 2"=→"Probe 2":fxp<+/-,16,16>, "Probe 3"=→"Probe 3":fxp<+/-,39,24>, "Probe 5"=→"Probe 5":fxp<+/-,16,2>, "Probe 7"=→"Probe 7":fxp<+/-,18,1>, "IProbe"=→"I Probes":T15, "Probe 21"=→"Probe 21":fxp<+/-,24,5>, "Probe 22"=→"Probe 22":fxp<+/-,54,35>, "Probe 23"=→"Probe 23":fxp<+/-,54,1>, "Probe 24"=→"Probe 24":fxp<+/-,16,1>, "Probe Offsetd"=→"Probe Offsetd":fxp<+/-,16,16>, "QProbe"=→"Q Probes":T15, "AI_Over"=w1102:bool, "10MHzLocked"=→"10 MHzPLL Status":bool)
        n503 = First Call?() -> (First Call?: T/F=w1104:bool)
        n504 = Select(t=6.0 ("Set Start Time (s)"), s=w1104, f=0.0) -> (s? t:f=w1105:dbl)
        n505 = call "Elapsed Time6"("Time Target (s)"=5.0, "Reset"=w1102, "Set Start Time (s)"=w1105) -> ("Time has Elapsed"=w1103:bool)  [unwired: 9 in, 7 out]
        n506 = Not(x=w1103) -> (.not. x?=→"Input Over Range":bool)
      }
      frame "FP_PXI" {
        n507 = Variant To Data(error in=w1135, type=T57 {"Temperatures"=[], "Fans"=[], "Voltages"=[]} ("PXI"), Variant=w1133) -> (data=w1131:T57, error out=w1134:errorcluster)
        n508 = Unbundle By Name(w1131) -> ("Temperatures"=→"Temperatures":string[][], "Fans"=→"Fans":string[][], "Voltages"=→"Voltages":string[][])
      }
      frame "FP_AI" {
        n509 = Variant To Data(error in=w1155, type=T58 {"AI"={"TimeString"="", "Time Stamp"=0.0, "AI0_Unused"=0.0, "AI1_-5V"=0.0, "AI2_+5V"=0.0, "AI3_+6V"=0.0, "AI4_+12V"=0.0, "AI5_+15V"=0.0, "AI6_+28V"=0.0, "AI7_Unused"=0.0, "Ai16_72GHz_CalPower"=0.0, "Ai17_84GHz_CalPower"=0.0, "Ai18_InclinAz"=0.0, "Ai19_InclinEl"=0.0, "Ai20_BlowerPwr"=0.0, "Ai21_Unused"=0.0, "Ai22_Unused"=0.0, "Ai23_Unused"=0.0, "InclinA_StdDev"=0.0, "InclinB_StdDev"=0.0, "InclinAz_Unfilt"=0.0, "InclinEl_Unfilt"=0.0}, "AllErrorStatus"={"AI 0"={"RX?"=FALSE, "Warn"=FALSE, "Error"=FALSE, "Enabl"=FALSE, "Source"=""}, "AI 1"={"RX?"=FALSE, "Warn"=FALSE, "Error"=FALSE, "Enabl"=FALSE, "Source"=""}, "AI 2"={"RX?"=FALSE, "Warn"=FALSE, "Error"=FALSE, "Enabl"=FALSE, "Source"=""}, "AI 3"={"RX?"=FALSE, "Warn"=FALSE, "Error"=FALSE, "Enabl"=FALSE, "Source"=""}, "AI 4"={"RX?"=FALSE, "Warn"=FALSE, "Error"=FALSE, "Enabl"=FALSE, "Source"=""}, "AI 5"={"RX?"=FALSE, "Warn"=FALSE, "Error"=FALSE, "Enabl"=FALSE, "Source"=""}, "AI 6"={"RX?"=FALSE, "Warn"=FALSE, "Error"=FALSE, "Enabl"=FALSE, "Source"=""}, "AI 7"={"RX?"=FALSE, "Warn"=FALSE, "Error"=FALSE, "Enabl"=FALSE, "Source"=""}, "AI 16"={"RX?"=FALSE, "Warn"=FALSE, "Error"=FALSE, "Enabl"=FALSE, "Source"=""}, "AI 17"={"RX?"=FALSE, "Warn"=FALSE, "Error"=FALSE, "Enabl"=FALSE, "Source"=""}, "AI 18"={"RX?"=FALSE, "Warn"=FALSE, "Error"=FALSE, "Enabl"=FALSE, "Source"=""}, "AI 19"={"RX?"=FALSE, "Warn"=FALSE, "Error"=FALSE, "Enabl"=FALSE, "Source"=""}, "AI 20"={"RX?"=FALSE, "Warn"=FALSE, "Error"=FALSE, "Enabl"=FALSE, "Source"=""}, "AI 21"={"RX?"=FALSE, "Warn"=FALSE, "Error"=FALSE, "Enabl"=FALSE, "Source"=""}, "AI 22"={"RX?"=FALSE, "Warn"=FALSE, "Error"=FALSE, "Enabl"=FALSE, "Source"=""}, "AI 23"={"RX?"=FALSE, "Warn"=FALSE, "Error"=FALSE, "Enabl"=FALSE, "Source"=""}}}, Variant=w1153) -> (data=w1151:T58, error out=w1154:errorcluster)
        n510 = Unbundle By Name(w1151) -> ("AI"=w1150:T59)
        n511 = call "SortVoltage_Display.vi"("Voltage"=w1150) -> ("VoltageDisplay"=w1145:T69)  [unwired: 10 in]
        n512 = Unbundle By Name(w1145) -> ("AI1_-5V"=→"-5V":dbl, "AI2_+5V"=→"+5":dbl, "AI3_+6V"=→"+6":dbl, "AI4_+12V"=→"+12":dbl, "AI5_+15V"=→"+15":dbl, "AI6_+28V"=→"+28":dbl, "Ai18_InclinometerAz"=→"InclAz":dbl, "Ai19_InclinometerEl"=→"InclEl":dbl, "Ai20_BlowerPower"=→"BlowerPower":dbl)  [unwired: 2 out]
        n513 = Unbundle By Name(w1145) -> ("Ai18_InclinometerAz"=w1149:dbl, "Ai19_InclinometerEl"=w1148:dbl)
        n514 = Bundle("Ai18_InclinometerAz"=w1149, "Ai19_InclinometerEl"=w1148) -> (→"Inclinometer History":T8)  [unwired: 1 in]
      }
      frame "FP_TC" {
